vi "Malleable VIs Basics Lesson 2.vi"() -> (3 "Last Numeric":dbl)   [LabVIEW 2017]
doc: "Learn how to create malleable VIs."
uses:
  f4955d1f-2e13-4bc1-a969-592dc4b69089.vi
panel:
  # "Overview: Learn how to create malleable VIs.\nInstructions: \n1. Complete the Lesson VIs prior to this one in the Malleable VIs Basics example project.\n2.  Open the block diagram of this VI. Review the lessons presented there.\n3. Once you have finished reviewing this VI, open the Lesson 3 VI in the Malleable VIs Basics example project."
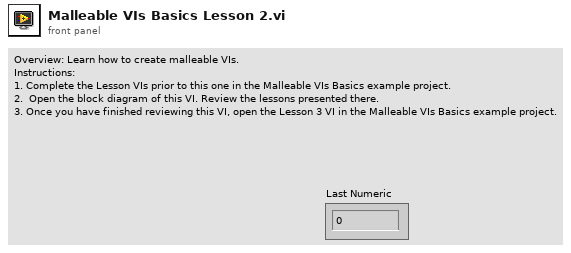
[diagram p1: front panel]
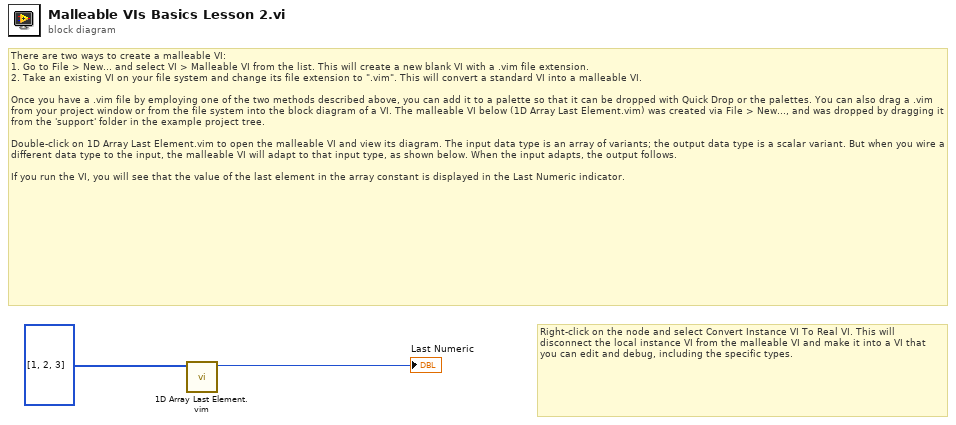
[diagram p0: block diagram]
diagram:
  # "Right-click on the node and select Convert Instance VI To Real VI. This will disconnect the local instance VI from the malleable VI and make it into a VI that you can edit and debug, including the specific types."
  # "There are two ways to create a malleable VI:\n1. Go to File > New... and select VI > Malleable VI from the list. This will create a new blank VI with a .vim file extension.\n2. Take an existing VI on your file system and change its file extension to \".vim\". This will convert a standard VI into a malleable VI.\n\nOnce you have a .vim file by employing one of the two methods described above, you can add it to a palette so that it can be dropped with Quick Drop or the palettes. You can also drag a .vim from your project window or from the file system into the block diagram of a VI. The malleable VI below (1D Array Last Element.vim) was created via File > New..., and was dropped by dragging it from the 'support' folder in the example project tree.\n\nDouble-click on 1D Array Last Element.vim to open the malleable VI and view its diagram. The input data type is an array of variants; the output data type is a scalar variant. But when you wire a different data type to the input, the malleable VI will adapt to that input type, as shown below. When the input adapts, the output follows.\n\nIf you run the VI, you will see that the value of the last element in the array constant is displayed in the Last Numeric indicator."
  n1 = call "1D Array Last Element.vim"("1D Array"=i32[] [1, 2, 3]) -> ("Last Element"=→"Last Numeric":i32)  [unwired: 10 in]
